vi "circulatingTheBall.vi"() -> ()   [LabVIEW 2021, in "KickToSkill.lvclass"]
uses:
  KickToSkill.lvclass
  Robot_class/Robot.lvclass
  Game_class/Game.lvclass
  Game_class/Game.lvclass/Game.ctl
  Object_class/Object.lvclass/Object.ctl
  Robot_class/Robot.lvclass/Robot.ctl
  <vilib>/Analysis/baseanly.llb/Unit Vector (DBL).vi
  <vilib>/Analysis/coordinate.llb/2D Cartesian Coordinate Rotation (Scalar).vi
  Object_class/Read position(x,y).vi
  Game_class/Read BallRef.vi
  Robot_class/Write dest_x.vi
  Robot_class/Write dest_y.vi
  Robot_class/Write dest_orientation.vi
  Robot_class/Write dribble.vi
  Robot_class/Write kick_x.vi
  Ball_class/Ball.lvclass
  <vilib>/Analysis/NI_AALPro.lvlib
  <vilib>/Analysis/NI_AALBase.lvlib
panel:
  out "Robot out":refnum<class "Robot.lvclass">
  in  "Raio":dbl=123.0
  in  "Game":refnum<class "Game.lvclass">
  in  "Target":dbl[](array[numeric])
  in  "Robot in":refnum<class "Robot.lvclass">
  out "KickToSkill out":refnum<class "KickToSkill.lvclass">
  in  "KickToSkill in":refnum<class "KickToSkill.lvclass">
  out "error out":errorcluster
  in  "error in (no error)":errorcluster
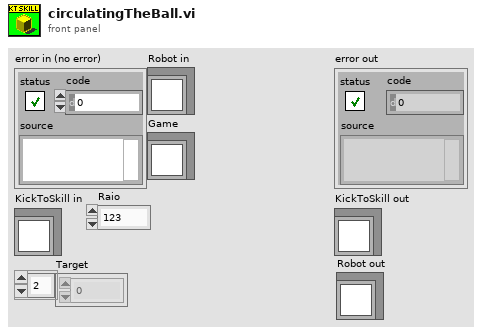
[diagram p1: front panel]
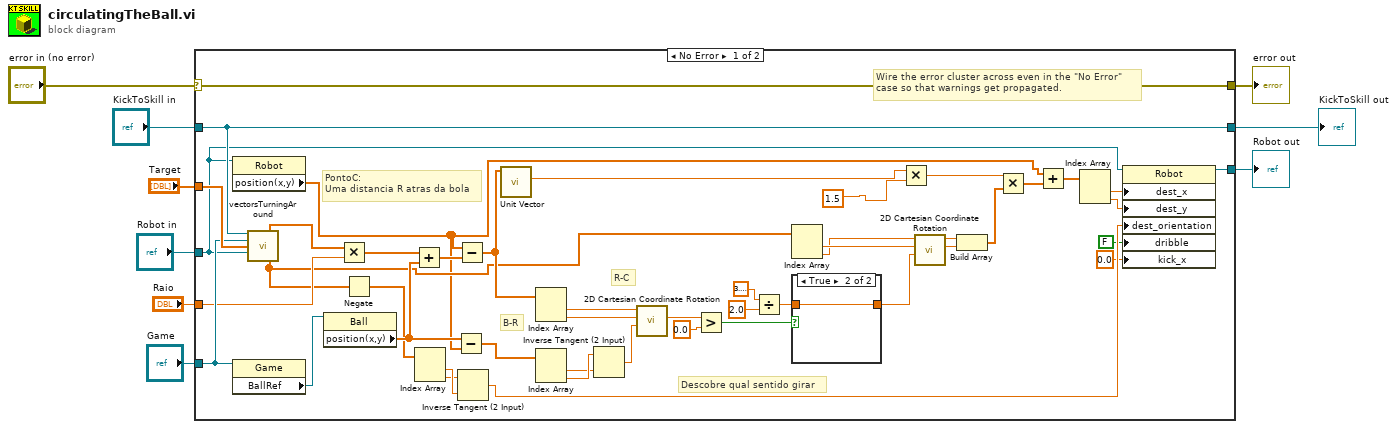
[diagram p0: block diagram]
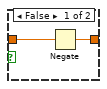
[diagram p2: hidden frame]
diagram:
  n1 = case shown="No Error" "error in (no error)" {
    selector: "error in (no error)" -> [w55 w61]
    tunnel: [w55 w61] -> w8
    tunnel: [w54 w60] -> w6
    tunnel: "KickToSkill in" -> [w54 w60]
    tunnel: "Game" -> [w51 _]
    tunnel: "Target" -> [w53 _]
    tunnel: "Robot in" -> [w28 w59]
    tunnel: [w52 w59] -> w2
    tunnel: "Raio" -> [w30 _]
    frame No Error {
      # "PontoC:\nUma distancia R atras da bola"
      # "B-R"
      # "R-C"
      # "Descobre qual sentido girar"
      # "Wire the error cluster across even in the \"No Error\"\ncase so that warnings get propagated."
      n2 = property class="Robot"(reference=w28) -> ("position(x,y)"=w12:dbl[])  [unwired: 1 in, 2 out]
      n3 = property class="Game"(reference=w51) -> ("BallRef"=w50:refnum<class "Ball.lvclass">)  [unwired: 1 in, 2 out]
      n4 = call "vectorsTurningAround.vi"("KickToSkill in"=w54, "Game"=w51, "Target"=w53, "Robot in"=w28) -> ("B-T"=w31:dbl[], "R-B"=w19:dbl[])  [unwired: 4 in, 6 out]
      n5 = property class="Ball"(reference=w50) -> ("position(x,y)"=w26:dbl[])  [unwired: 1 in, 2 out]
      n6 = Multiply(x=w31, y=w30) -> (x*y=w29:dbl[])
      n7 = Negate(x=w19) -> (-x=w18:dbl[])
      n8 = Add(x=w29, y=w26) -> (x+y=w25:dbl[])
      n9 = Index Array(array=w18) -> (element #1=w17:dbl, element #2=w16:dbl)  [unwired: 2 in]
      n10 = Subtract(x=w26, y=w12) -> (x-y=w24:dbl[])
      n11 = Subtract(x=w12, y=w25) -> (x-y=w27:dbl[])
      n12 = Inverse Tangent (2 Input)(1:w17, 2:w16) -> (0:w49:dbl)
      n13 = call-poly <vilib>:"Unit Vector.vi"("Input Vector"=w27) -> ("norm"=w15:dbl)  [unwired: 8 in, 2 out]
      n14 = Index Array(array=w27) -> (element #1=w42:dbl, element #2=w41:dbl)  [unwired: 2 in]
      n15 = Index Array(array=w24) -> (element #1=w35:dbl, element #2=w36:dbl)  [unwired: 2 in]
      n16 = Inverse Tangent (2 Input)(1:w35, 2:w36) -> (0:w40:dbl)
      n17 = call-poly <vilib>:"2D Cartesian Coordinate Rotation.vi"("theta"=w40, "y"=w41, "x"=w42) -> ("y out"=w39:dbl)  [unwired: 6 in, 2 out]
      n18 = Greater?(x=w39, y=0.0) -> (0:w37:bool)
      n19 = Divide(x=3.141592653589793, y=2.0) -> (x/y=w44:dbl)
      n20 = Index Array(array=w19) -> (element #1=w23:dbl, element #2=w22:dbl)  [unwired: 2 in]
      n21 = case shown="True" w37 {
        tunnel: w44 -> [w57 w58]
        tunnel: [w56 w58] -> w43
        frame False {
          n22 = Negate(x=w57) -> (-x=w56:dbl)
        }
        frame True {
        }
      }
      n23 = Multiply(x=w15, y=1.5) -> (x*y=w14:dbl)
      n24 = call-poly <vilib>:"2D Cartesian Coordinate Rotation.vi"("theta"=w43, "y"=w23, "x"=w22) -> ("y out"=w47:dbl, "x out"=w48:dbl)  [unwired: 6 in, 1 out]
      n25 = Build Array(w48, w47) -> (w34:dbl[])
      n26 = Multiply(x=w14, y=w34) -> (x*y=w33:dbl[])
      n27 = Add(x=w12, y=w33) -> (x+y=w32:dbl[])
      n28 = Index Array(array=w32) -> (element #1=w21:dbl, element #2=w20:dbl)  [unwired: 2 in]
      n29 = property class="Robot"(reference=w28, "dest_x"=w21, "dest_y"=w20, "dest_orientation"=w49, "dribble"=FALSE, "kick_x"=0.0) -> (reference out=w52:refnum<class "Robot.lvclass">)  [unwired: 1 in, 1 out]
    }
    frame Error {
    }
  }
  "error out" <- w8
  "KickToSkill out" <- w6
  "Robot out" <- w2
